vi "Set Ctl Value.vi"(8 "error in (no error)":errorcluster, 9 "Signaling?":bool, 10 "String":string, 11 "Text field in":refnum<class "Text field.lvclass">) -> (0 "error out":errorcluster, 3 "Text field out":refnum<class "Text field.lvclass">)   [LabVIEW 2020, in "Text field.lvclass"]
uses:
  Text field.lvclass
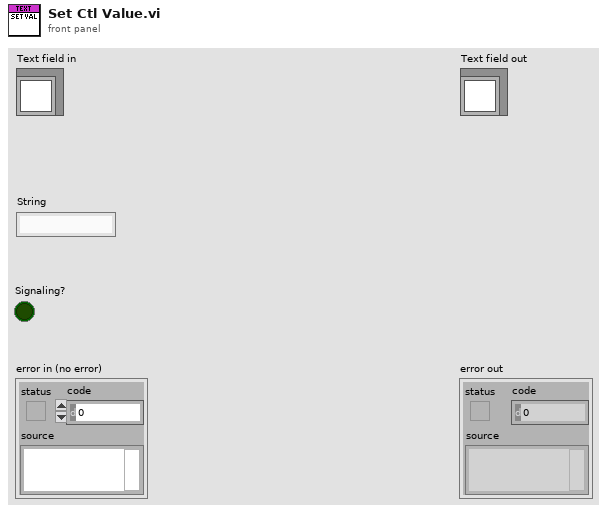
[diagram p1: front panel]
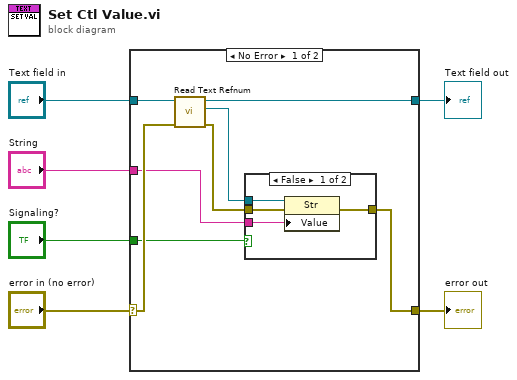
[diagram p0: block diagram]
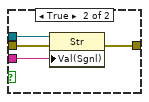
[diagram p2: hidden frame]
diagram:
  n1 = case shown="No Error" "error in (no error)" {
    selector: "error in (no error)" -> [w12 w24]
    tunnel: [w7 w24] -> w5
    tunnel: "Text field in" -> [w14 w23]
    tunnel: [w13 w23] -> w3
    tunnel: "Signaling?" -> [w10 _]
    tunnel: "String" -> [w9 _]
    frame No Error {
      n2 = call "Read Text Refnum.vi"("error in (no error)"=w12, "Text field in"=w14) -> ("error out"=w8:errorcluster, "Str Refnum"=w11:refnum<vi>, "Text field out"=w13:refnum<class "Text field.lvclass">)  [unwired: 7 in]
      n3 = case shown="False" w10 {
        tunnel: w11 -> [w18 w22]
        tunnel: w9 -> [w16 w21]
        tunnel: w8 -> [w17 w20]
        tunnel: [w15 w19] -> w7
        frame False {
          n4 = property class="Str"(reference=w18, error in=w17, "Value"=w16) -> (error out=w15:errorcluster)  [unwired: 1 out]
        }
        frame True {
          n5 = property class="Str"(reference=w22, error in=w20, "Val(Sgnl)"=w21) -> (error out=w19:errorcluster)  [unwired: 1 out]
        }
      }
    }
    frame Error {
    }
  }
  "error out" <- w5
  "Text field out" <- w3
